vi "myRIO_BRig_RT_dataLC_Reward_Trial_l1.vi"() -> (2 "output_Reward_Trial_l1":i32)   [LabVIEW 2014]
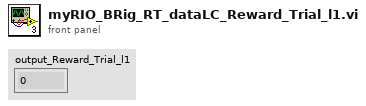
[diagram p1: front panel]
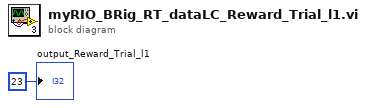
[diagram p0: block diagram]
diagram:
  "output_Reward_Trial_l1" <- 23 ("output_iBlock")
